vi "Obtain Hwnd-LV RT.vi"(0 "LV RT in":refnum<class "LV RT.lvclass">, 11 "error in (no error)":errorcluster) -> (4 "LV RT out":refnum<class "LV RT.lvclass">, 15 "error out":errorcluster)   [LabVIEW 2016, in "LV RT.lvclass"]
uses:
  LV RT.lvclass
  D:/MDI Project/source code/Document/Child Classes/LV Doc/LV Doc.lvclass
  D:/MDI Project/source code/Document/Document.lvclass
  LV Doc.lvclass/LV Doc.ctl
  Document.lvclass/Document.ctl
  LV Doc.lvclass
  Document.lvclass
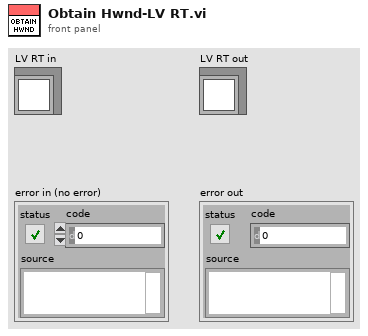
[diagram p1: front panel]
types:
  T1 = enum32{"Invalid", "Standard", "Closed", "Hidden", "Minimized", "Maximized"}
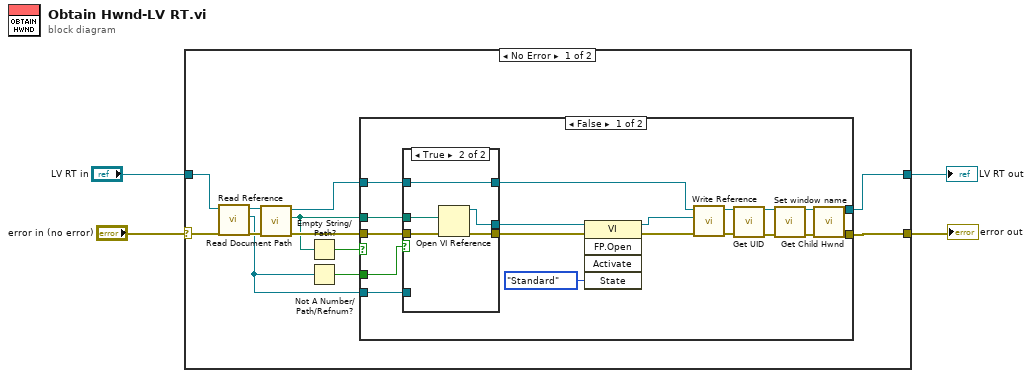
[diagram p0: block diagram]
diagram:
  n1 = case shown="No Error" "error in (no error)" {
    selector: "error in (no error)" -> [w12 w46]
    tunnel: [w16 w47] -> w4
    tunnel: [w15 w46] -> w3
    tunnel: "LV RT in" -> [w10 w47]
    frame No Error {
      n2 = call "Read Reference.vi"("error in (no error)"=w12, "LV Doc in"=w10) -> ("error out"=w11:errorcluster, "Reference"=w8:refnum<vi>, "LV Doc out"=w9:refnum<class "LV RT.lvclass">)  [unwired: 7 in]
      n3 = call "Read Document Path.vi"("error in (no error)"=w11, "Document in"=w9) -> ("error out"=w13:errorcluster, "Document Path"=w6:path, "Document out"=w14:refnum<class "LV RT.lvclass">)  [unwired: 7 in]
      n4 = Empty String/Path?(string/path=w6) -> (empty?=w5:bool)
      n5 = Not A Number/Path/Refnum?(number/path/refnum=w8) -> (NaN/Path/Refnum?=w7:bool)
      n6 = case shown="False" w5 {
        tunnel: [w35 w45] -> w16
        tunnel: [w34 w44] -> w15
        tunnel: w14 -> [w33 w45]
        tunnel: w13 -> [w32 w44]
        tunnel: w6 -> [w31 _]
        tunnel: w8 -> [w30 _]
        tunnel: w7 -> [w17 _]
        frame False {
          n7 = case shown="True" w17 {
            tunnel: [w37 w43] -> w21
            tunnel: [w38 w42] -> w20
            tunnel: w32 -> [w38 w41]
            tunnel: w31 -> [_ w40]
            tunnel: w30 -> [w37 _]
            tunnel: w33 -> [w36 w39]
            tunnel: [w36 w39] -> w19
            frame False {
            }
            frame True {
              n8 = Open VI Reference(vi path=w40, error in (no error)=w41) -> (vi reference=w43:refnum<vi>, error out=w42:errorcluster)  [unwired: 4 in]
            }
          }
          n9 = invoke class="VI" method="FP.Open"(reference=w21, error in=w20, "State"=T1."Standard") -> (reference out=w23:refnum<vi>, error out=w18:errorcluster)  [unwired: 2 in, 3 out]
          n10 = call "Write Reference.vi"("error in (no error)"=w18, "Reference"=w23, "LV Doc in"=w19) -> ("error out"=w26:errorcluster, "LV Doc out"=w27:refnum<class "LV RT.lvclass">)  [unwired: 7 in]
          n11 = call "Get UID.vi"("LV Doc.lvclass"=w27, "error in (no error)"=w26) -> ("LV Doc.lvclass"=w25:refnum<class "LV RT.lvclass">, "error out"=w28:errorcluster)  [unwired: 12 in]
          n12 = call "Set window name.vi"("LV Doc.lvclass"=w25, "error in (no error)"=w28) -> ("LV Doc.lvclass"=w24:refnum<class "LV RT.lvclass">, "error out"=w29:errorcluster)  [unwired: 12 in]
          n13 = call "Get Child Hwnd.vi"("LV Doc.lvclass"=w24, "Error in"=w29) -> ("LV Doc.lvclass"=w35:refnum<class "LV RT.lvclass">, "Error Out"=w34:errorcluster)  [unwired: 12 in]
        }
        frame True {
        }
      }
    }
    frame Error {
    }
  }
  "LV RT out" <- w4
  "error out" <- w3
